vi "move_galvo_trigger.vi"(0 "TAG trigger":bool) -> (1 "counts in last cycle":u16, 2 "split trigger":bool)   [LabVIEW 2010]
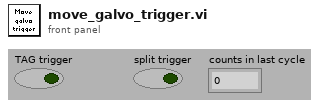
[diagram p1: front panel]
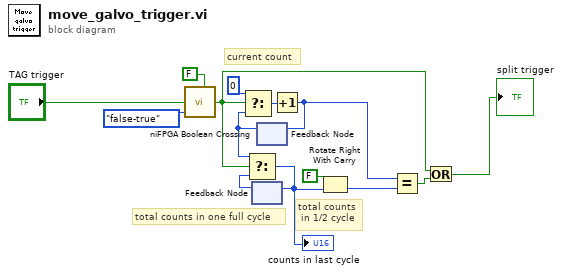
[diagram p0: block diagram]
diagram:
  # "total counts\n in 1/2 cycle"
  # "total counts in one full cycle"
  # "current count"
  n1 = call <vilib>:"niFPGA Boolean Crossing.vi"("input"="TAG trigger", "direction"=enum8{"either", "false-true", "true-false"}."false-true", "initialize"=FALSE) -> ("crossing"=w2:bool)  [unwired: 6 in]
  n2 = feedback #1() -> (w8:u16)  [unwired: 1 in]
  n3 = feedback #2() -> (w7:u16)  [unwired: 1 in]
  n4 = Select(t=u16 0, s=w2, f=w7) -> (s? t:f=w11:u16)
  n5 = Select(t=w7, s=w2, f=w8) -> (s? t:f=w10:u16)
  "counts in last cycle" <- w10
  n6 = feedback-in #1(w10) -> ()
  n7 = Increment(x=w11) -> (x+1=w13:u16)
  n8 = feedback-in #2(w13) -> ()
  n9 = Rotate Right With Carry(2:w10, 3:FALSE ("carry")) -> (0:w14:u16)  [unwired: 1 out]
  n10 = Equal?(x=w13, y=w14) -> (x = y?=w3:bool)
  n11 = Or(x=w2, y=w3) -> (x .or. y?=→"split trigger":bool)
